vi "database.vi"(11 "db file":path=path "E:/backup/FACE_images/Set2/OneDrive_2020-09-29/ST100242 FACEv2 pilot/DB/ST100242.db") -> (2 "viewid":string[](array[string]), 3 "filepath":path[](array[path]))   [LabVIEW 2024]
uses:
  <vilib>/drjdpowell/SQLite Library/SQL Statement/SQL Statement.lvclass/SQL Statement.ctl
  <vilib>/drjdpowell/SQLite Library/SQL Connection/Open (path).vi
  <vilib>/drjdpowell/SQLite Library/SQL Statement/Bind Text.vi
  <vilib>/drjdpowell/SQLite Library/SQL Connection/Open (string).vi
  <vilib>/AdvancedString/Path To Command Line String.vi
  <vilib>/drjdpowell/SQLite Library/SQL Statement/Error Message.vi
  <vilib>/drjdpowell/SQLite Library/SQL Statement/Column String.vi
  <vilib>/drjdpowell/SQLite Library/SQL Connection/Connection.lvclass
  <vilib>/drjdpowell/SQLite Library/SQL Statement/SQL Statement.lvclass
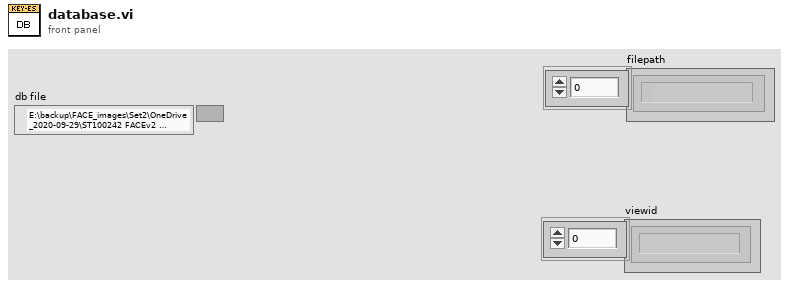
[diagram p1: front panel]
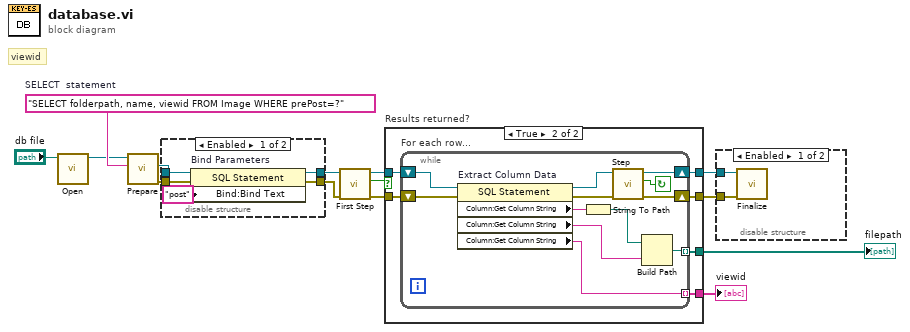
[diagram p0: block diagram]
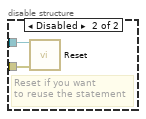
[diagram p2: hidden frame]
diagram:
  w12 = "SELECT folderpath, name, viewid FROM Image WHERE prePost=?"  # SELECT  statement
  # "viewid"
  n1 = call-poly <vilib>:"Open.vi"("db file"="db file") -> ("SQLite Connection"=w4:refnum<class "Connection.lvclass">)  [unwired: 9 in, 1 out]
  n2 = call <vilib>:"Prepare.vi"("SQL"=w12, "SQLite Connection in"=w4) -> ("error out"=w11:errorcluster, "SQL Statement"=w8:refnum<class "SQL Statement.lvclass">)  [unwired: 5 in, 3 out]
  n3 = disable-structure shown="Enabled" {
    disable-tunnel: w8 -> [w19 w21]
    disable-tunnel: [w18 w21] -> w9
    disable-tunnel: [w17 w20] -> w10
    disable-tunnel: w11 -> [w16 w20]
    frame Enabled {
      n4 = property on="Bind Parameters" class="SQL Statement"(reference=w19, error in=w16, "Bind:Bind Text"="post" ("Bind:Text")) -> (reference out=w18:refnum<class "SQL Statement.lvclass">, error out=w17:errorcluster)
    }
    frame Disabled {
    }
  }
  n5 = call <vilib>:"First Step.vi"("error in (no error)"=w10, "SQL Statement in"=w9) -> ("error out"=w6:errorcluster, "Row returned"=w5:bool, "SQL Statement"=w7:refnum<class "SQL Statement.lvclass">)  [unwired: 7 in]
  n6 = case "Results returned?" shown="True" w5 {
    tunnel: [w23 w29] -> w13
    tunnel: [w22 w28] -> w14
    tunnel: w7 -> [w23 w27]
    tunnel: w6 -> [w22 w26]
    tunnel: [_ w25] -> w1
    tunnel: [_ w24] -> w2
    frame False {
    }
    frame True {
      n7 = while "For each row..." {
        shift-right: [w40] -> w29
        shift-left: w27 -> [w37]
        shift-right: [w38] -> w28
        shift-left: w26 -> [w36]
        tunnel: [w30] -> w25 mode=indexing
        tunnel: [w34] -> w24 mode=indexing
        stop <- w35 continue-if-true
        n8 = property on="Extract Column Data" class="SQL Statement"(reference=w37, error in=w36) -> (reference out=w41:refnum<class "SQL Statement.lvclass">, error out=w39:errorcluster, "Column:Get Column String"=w33:string, "Column:Get Column String"=w31:string, "Column:Get Column String"=w34:string)
        n9 = String To Path(string=w33) -> (path=w32:path)
        n10 = call <vilib>:"Step.vi"("error in (no error)"=w39, "SQL Statement in"=w41) -> ("error out"=w38:errorcluster, "Row returned"=w35:bool, "SQL Statement"=w40:refnum<class "SQL Statement.lvclass">)  [unwired: 7 in]
        n11 = Build Path(base path=w32, name or relative path=w31) -> (appended path=w30:path)
      }
    }
  }
  "viewid" <- w2
  "filepath" <- w1
  n12 = disable-structure shown="Enabled" {
    disable-tunnel: w13 -> [w43 w45]
    disable-tunnel: w14 -> [w42 w44]
    frame Enabled {
      n13 = call <vilib>:"Finalize.vi"("error in (no error)"=w42, "SQL Statement in"=w43) -> ()  [unwired: 9 in, 1 out]
    }
    frame Disabled {
      # "Reset if you want\nto reuse the statement"
      n14 = call <vilib>:"Reset.vi"("error in (no error)"=w44, "SQL Statement in"=w45) -> ()  [unwired: 8 in, 2 out]
    }
  }
